vi "ArrayToExcel.vi"() -> ()   [LabVIEW 2020]
uses:
  <vilib>/Analysis/NI_AALBase.lvlib
panel:
  out "Tabla":string[][](array[string])
  out "Gráfica":dbl[][](graph)
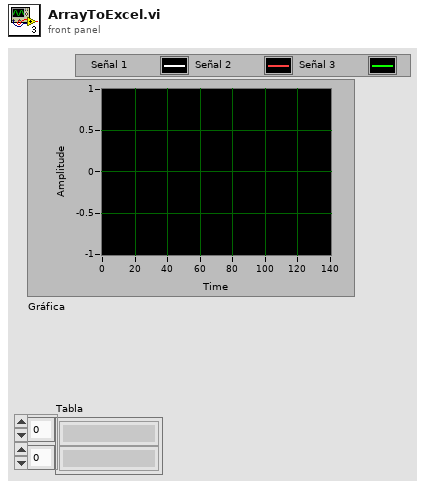
[diagram p1: front panel]
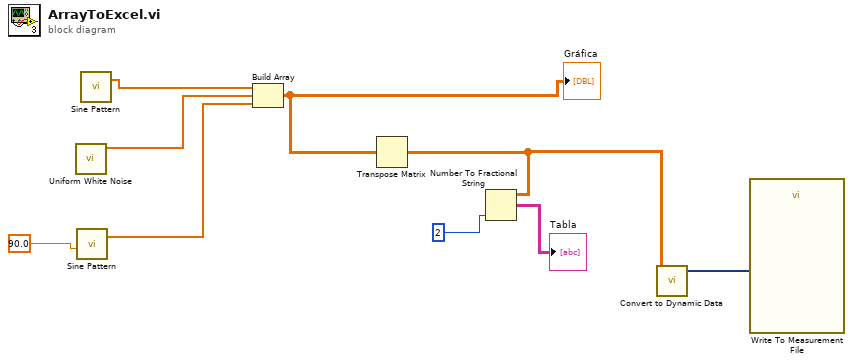
[diagram p0: block diagram]
diagram:
  n1 = call <vilib>:"Uniform White Noise.vi"() -> ("uniform white noise"=w7:dbl[])  [unwired: 10 in, 1 out]
  n2 = call <vilib>:"Sine Pattern.vi"("phase(degrees)"=90.0) -> ("Sinusoidal Pattern"=w6:dbl[])  [unwired: 3 in, 1 out]
  n3 = call <vilib>:"Sine Pattern.vi"() -> ("Sinusoidal Pattern"=w8:dbl[])  [unwired: 4 in, 1 out]
  n4 = Build Array(w8, w7, w6) -> (w5:dbl[][])
  "Gráfica" <- w5
  n5 = Transpose Matrix(1:w5) -> (0:w3:dbl[][])
  n6 = Number To Fractional String(number=w3, precision (6)=2) -> (F-format string=→"Tabla":string[][])  [unwired: 2 in]
  n7 = call "Convert to Dynamic Data"("2D Array"=w3) -> ("Dynamic Data Type"=w4:dynamicdata)  [unwired: 3 in]
  n8 = call "Write To Measurement File"("Signals"=w4) -> ()  [unwired: 16 in, 3 out]
